vi "FGV User Details.vi"(8 "error in":errorcluster, 10 "User Details":T1, 11 "Action":enum16{"Initialize", "Read", "Write"}(ring)) -> (0 "error out":errorcluster, 3 "User Details out":T1)   [LabVIEW 2019]
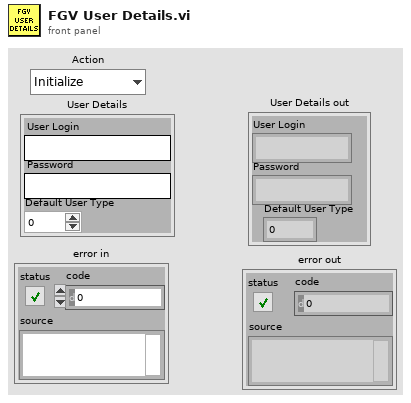
[diagram p1: front panel]
types:
  T1 = cluster{"User Login":string, "Password":string, "Default User Type":u16}
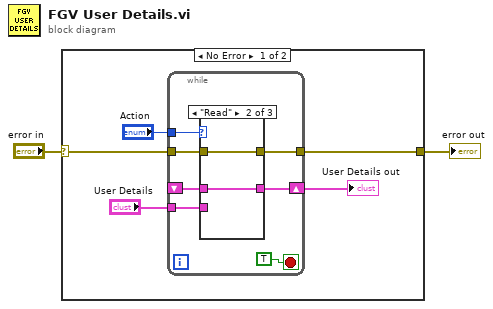
[diagram p0: block diagram]
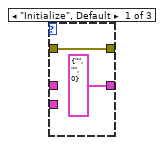
[diagram p2: hidden frame]
diagram:
  n1 = case shown="No Error" "error in" {
    selector: "error in" -> [w4 w21]
    tunnel: [w3 w21] -> w1
    frame No Error {
      n2 = while {
        tunnel: "Action" -> [w14]
        shift-right: [w12] -> w5
        shift-left: _ -> [w11]
        tunnel: "User Details" -> [w13]
        tunnel: w4 -> [w9]
        tunnel: [w8] -> w3
        stop <- TRUE stop-if-true
        n3 = case shown="\"Read\"" w14 {
          tunnel: w13 -> [_ _ w20]
          tunnel: [T1 {"User Login"="", "Password"="", "Default User Type"=0} ("User Details") w18 w20] -> w12
          tunnel: w11 -> [_ w18 _]
          tunnel: [w15 w17 w19] -> w8
          tunnel: w9 -> [w15 w17 w19]
          frame "Initialize", Default {
          }
          frame "Read" {
          }
          frame "Write" {
          }
        }
      }
      "User Details out" <- w5
    }
    frame Error {
    }
  }
  "error out" <- w1
